vi "Initialize.vi"(8 "error in (no error)":errorcluster, 11 "UDP Configuration in":refnum<class "UDP Configuration.lvclass">) -> (0 "error out":errorcluster, 3 "UDP Configuration out":refnum<class "UDP Configuration.lvclass">)   [LabVIEW 2017, in "DSF Core.lvlib" / "UDP Configuration.lvclass"]
uses:
  UDP Configuration.lvclass
  C:/Git/DSF/Core/Classes/Component Configuration/Component Configuration.lvclass
  Classes/Configuration/Configuration.lvclass
  UDP Thread Configuration.lvclass
  C:/Git/DSF/Core/Classes/Configuration/Configuration.lvclass
  Classes/Component Configuration/Component Configuration.lvclass
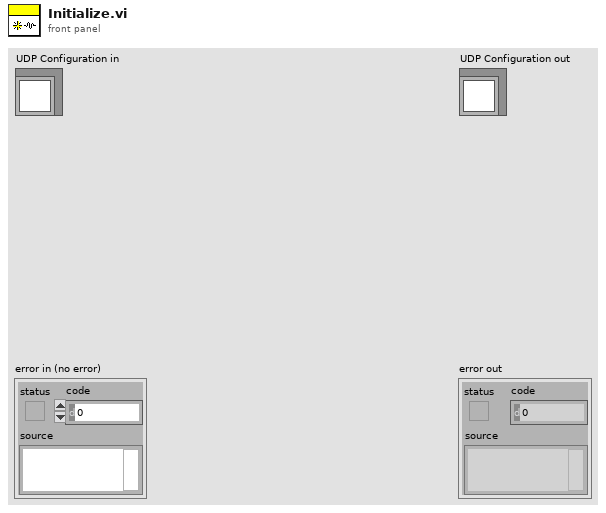
[diagram p1: front panel]
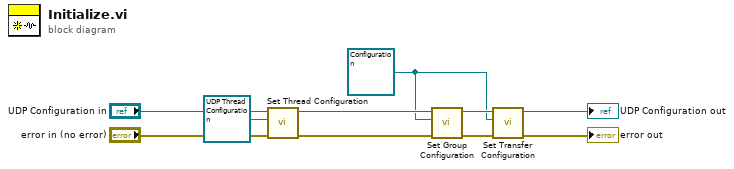
[diagram p0: block diagram]
diagram:
  w2 = refnum<class "Configuration.lvclass"> refnum ("Group Configuration")
  n1 = call "Set Thread Configuration.vi"("error in (no error)"="error in (no error)", "Thread Configuration"=refnum<class "UDP Thread Configuration.lvclass"> refnum ("DSF Core.lvlib:DSF UDP Thread Configuration"), "Component Configuration in"="UDP Configuration in") -> ("error out"=w7:errorcluster, "Component Configuration out"=w8:refnum<class "UDP Configuration.lvclass">)  [unwired: 7 in]
  n2 = call "Set Group Configuration.vi"("error in (no error)"=w7, "Group Configuration"=w2, "Component Configuration in"=w8) -> ("error out"=w5:errorcluster, "Component Configuration out"=w6:refnum<class "UDP Configuration.lvclass">)  [unwired: 7 in]
  n3 = call "Set Transfer Configuration.vi"("error in (no error)"=w5, "Transfer Configuration"=w2, "Component Configuration in"=w6) -> ("error out"=→"error out":errorcluster, "Component Configuration out"=→"UDP Configuration out":refnum<class "UDP Configuration.lvclass">)  [unwired: 7 in]
